vi "Write Single Register.vi"(6 "timeout ms (1000)":i32=1000, 8 "error in (no error)":errorcluster, 9 "Value":u16, 10 "Address":u16, 11 "Modbus TCP Micro Master in":refnum<class "Modbus TCP Micro Master.lvclass">) -> (0 "error out":errorcluster, 3 "Modbus TCP Micro Master out":refnum<class "Modbus TCP Micro Master.lvclass">)   [LabVIEW 2023, in "Modbus TCP Micro.lvlib" / "Modbus TCP Micro Master.lvclass"]
uses:
  Modbus TCP Micro Master.lvclass
  Modbus TCP Micro Master.lvclass/Modbus TCP Micro Master.ctl
  Raw/Modbus Request.vi
  Modbus TCP Micro.lvlib
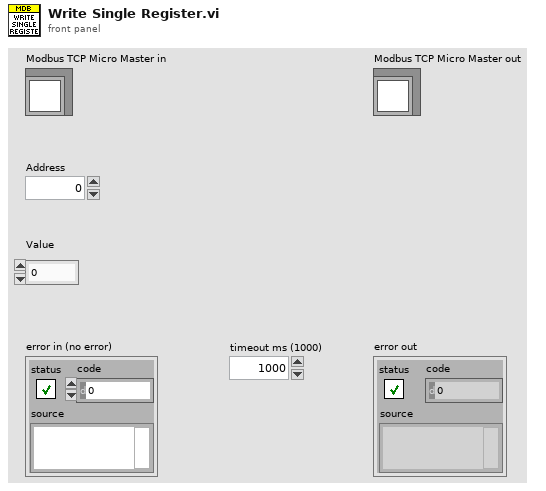
[diagram p1: front panel]
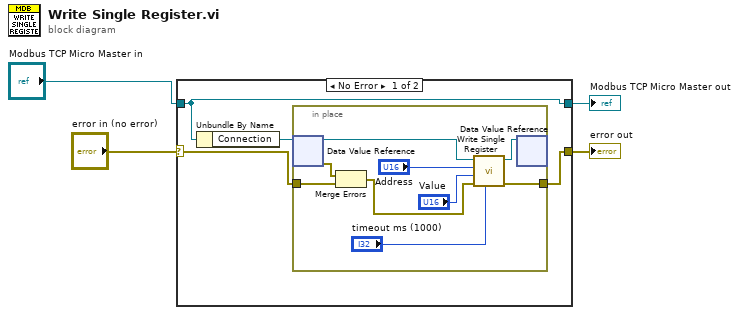
[diagram p0: block diagram]
diagram:
  n1 = case shown="No Error" "error in (no error)" {
    selector: "error in (no error)" -> [w6 w19]
    tunnel: [w5 w19] -> w3
    tunnel: [w8 w18] -> w1
    tunnel: "Modbus TCP Micro Master in" -> [w8 w18]
    frame No Error {
      n2 = Unbundle By Name(w8) -> ("Connection"=w7:refnum<data-value>)
      n3 = in-place {
        in-place-border: w6 -> [w17]
        in-place-border: [w16] -> w5
        n4 = in-place-dvr #1(w7) -> (w15:refnum<k5>, w12:errorcluster)
        n5 = Merge Errors(w12, w17) -> (w13:errorcluster)
        n6 = call "Write Single Register.vi"("timeout ms (1000)"="timeout ms (1000)", "error in (no error)"=w13, "Value"="Value", "Address"="Address", "TCP Network Connection in"=w15) -> ("error out"=w16:errorcluster, "TCP Network Connection out"=w14:refnum<k5>)  [unwired: 5 in]
        n7 = in-place-dvr #1(w14) -> ()  [unwired: 2 out]
      }
    }
    frame Error {
    }
  }
  "error out" <- w3
  "Modbus TCP Micro Master out" <- w1
